vi "Read Time.vi"(11 "Simple Actor in":refnum<class "Simple Actor.lvclass">) -> (2 "Time":dbl, 3 "Simple Actor out":refnum<class "Simple Actor.lvclass">)   [LabVIEW 2012, in "Simple Actor.lvclass"]
uses:
  Simple Actor.lvclass
  Simple Actor.lvclass/Simple Actor.ctl
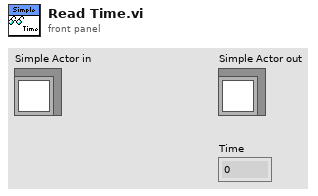
[diagram p1: front panel]
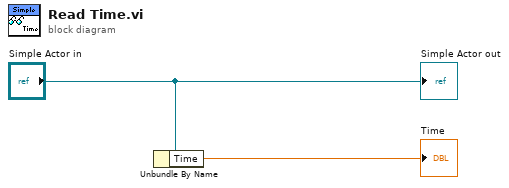
[diagram p0: block diagram]
diagram:
  n1 = Unbundle By Name("Simple Actor in") -> ("Time"=→"Time":dbl)
  "Simple Actor out" <- "Simple Actor in"
